vi "Initialize.vi"(6 "Start Direction":T1=enum."E", 8 "error in (no error)":errorcluster, 9 "Kamikaze DVR":T2, 10 "SquareStatus DVR":T3, 11 "Protector in":refnum<class "Protector.lvclass">) -> (0 "error out":errorcluster, 3 "Protector out":refnum<class "Protector.lvclass">)   [LabVIEW 2014, in "Protector.lvclass"]
uses:
  Protector.lvclass
  Mother/SquareStatus DVR.ctl
  Mother/Kamikaze DVR.ctl
  Direction Enum.ctl
  Protector.lvclass/Protector.ctl
  Mother/Mother.lvclass
  SquareBattle.lvclass
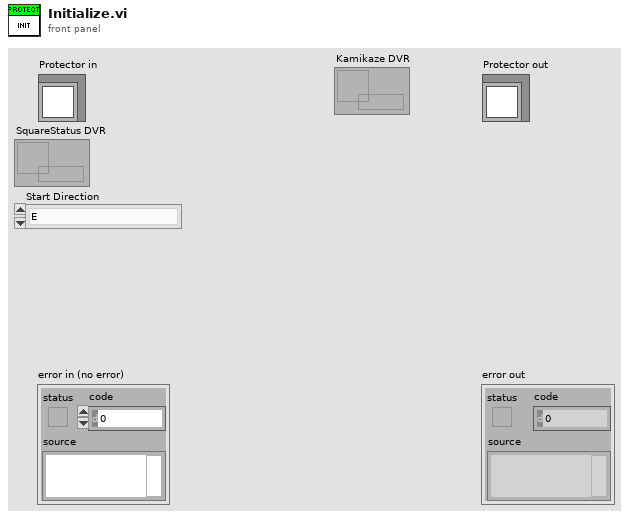
[diagram p1: front panel]
types:
  T1 = typedef "SquareBattle.lvclass/Direction Enum.ctl" = enum16{"NW", "N", "NE", "E", "SE", "S", "SW", "W"}
  T2 = typedef "Mother.lvclass/Kamikaze DVR.ctl" = refnum<data-value>
  T3 = typedef "Mother.lvclass/SquareStatus DVR.ctl" = refnum<data-value>
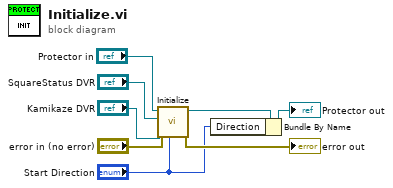
[diagram p0: block diagram]
diagram:
  n1 = call-parent "Initialize.vi"("Start Direction"="Start Direction", "error in (no error)"="error in (no error)", "Kamikaze DVR"="Kamikaze DVR", "SquareStatus DVR"="SquareStatus DVR", "Mother in"="Protector in") -> ("error out"=→"error out":errorcluster, "Mother out"=w7:refnum<class "Protector.lvclass">)  [unwired: 5 in]
  n2 = Bundle By Name(cluster=w7, "Direction"="Start Direction") -> (→"Protector out":refnum<class "Protector.lvclass">)
